vi "AutonomousChoose Postion.vi"() -> ()   [LabVIEW 2017]
doc: "This VI starts when autonomous period begins, and will automatically be terminated when it ends. You can carry out timed or sensor driven operations directly to I/O or to subsystems without needing to return to the caller."
uses:
  <vilib>/Rock Robotics/Network Tables/NT Read String.vi
panel:
  out "HandsMotorCmd":dbl(graph)
  out "Waveform Chart 4":u32(graph)
  out "millisecond timer value 2":u32
  out "SqueezeMotorCmd":dbl(graph)
  out "Lift Min Limit":bool
  out "Lift Max Limit":bool
  out "LiftMotorCmd":dbl(graph)
  out "Left Arm Max Limit":bool
  out "Right Arm Max Limit":bool
  out "Right Arm Min Limit":bool
  out "Left Arm Min Limit":bool
  out "LeftArmMotorCmd":dbl(graph)
  out "RightArmMotorCmd":dbl(graph)
  out "Arm Lift Min Limit":bool
  out "Arm Lift Max Limit":bool
  out "ArmLiftMotorCmd":dbl(graph)
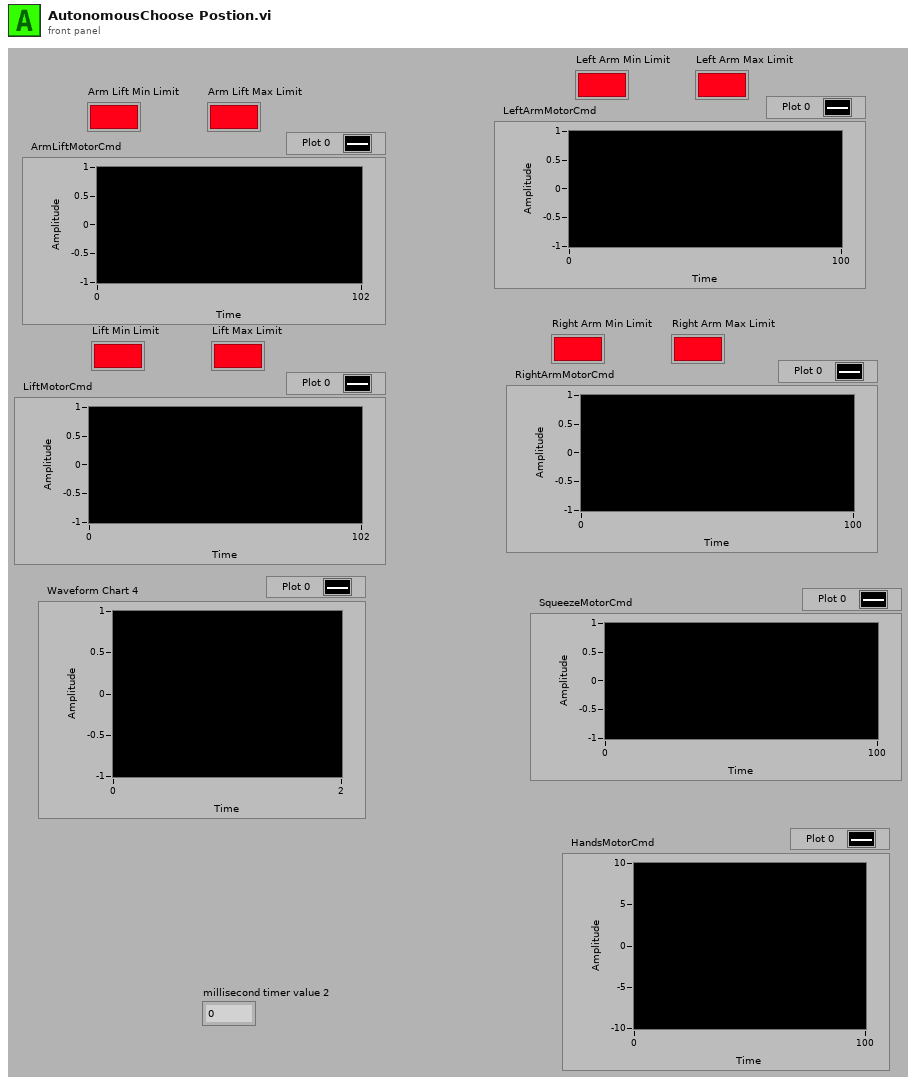
[diagram p1: front panel]
types:
  T1 = cluster{"X_axis":dbl, "Y_axis":dbl, "RotationTarget":dbl, "ArmLift":dbl, "Hands":dbl, "Lift":dbl, "Arms":dbl, "Squeeze":dbl}
  T2 = enum16{"initialize", "read", "write", "write all"}
  T3 = typedef "DioDisplayALB.ctl" = cluster{"DIO 0-LiftMinLimitSwitch":bool, "DIO 1-LiftMaxLimitSwitch":bool, "DIO 2-LiftArmMinLimitSwitch":bool, "DIO 3-LiftArmMaxLimitSwitch":bool, "DIO 4-RightArmMaxLimitSwitch":bool, "DIO 5-RightArmMinLimitSwitch":bool, "DIO 6-LeftArmMaxLimitSwitch":bool, "DIO 7-LeftArmMinLimitSwitch":bool, "DIO 8":bool, "DIO 9":bool}
  T4 = typedef "WPI_MotorControlDeviceRef.ctl" = cluster{"DeviceStatus":errorcluster, "Type":T5, "PWM":cluster{"PWM Channel":T6, "DeadBand":T7}, "CAN":cluster{"Device Number":u8, "SetOutput VI Ref":variant, "GetOutput VI Ref":variant, "Enable VI Ref":variant, "Disable VI Ref":variant, "Data":variant}, "Invert":bool, "DIO PWM":cluster{"PWM \"Enable\" Channel":T6, "DIOChannel":T8, "PWM Rate":dbl}}
  T5 = typedef "WPI_MotorControlType.ctl" = enum16{"PWM", "CAN", "DIO PWM"}
  T6 = typedef "FPGA_DIOPWMChannel.ctl" = enum8{"PWM 0", "PWM 1", "PWM 2", "PWM 3", "PWM 4", "PWM 5", "PWM 6", "PWM 7", "PWM 8", "PWM 9", "PWM MXP 0", "PWM MXP 1", "PWM MXP 2", "PWM MXP 3", "PWM MXP 4", "PWM MXP 5", "PWM MXP 6", "PWM MXP 7", "PWM MXP 8", "PWM MXP 9", "Invalid"}
  T7 = typedef "WPI_PWMDeadband.ctl" = cluster{"Name":string, "maxPositivePwm":i32, "minPositivePwm":i32, "centerPwm":i32, "maxNegativePwm":i32, "minNegativePwm":i32, "angularRange":u16}
  T8 = typedef "FPGA_DIOChannel.ctl" = enum8{"DIO 0", "DIO 1", "DIO 2", "DIO 3", "DIO 4", "DIO 5", "DIO 6", "DIO 7", "DIO 8", "DIO 9", "DIO MXP 0", "DIO MXP 1", "DIO MXP 2", "DIO MXP 3", "DIO MXP 4", "DIO MXP 5", "DIO MXP 6", "DIO MXP 7", "DIO MXP 8", "DIO MXP 9", "DIO MXP 10", "DIO MXP 11", "DIO MXP 12", "DIO MXP 13", "DIO MXP 14", "DIO MXP 15", "SPI Port CS1", "SPI Port CS2", "SPI Port CS3", "SPI Port MISO", "SPI Port MOSI", "Invalid"}
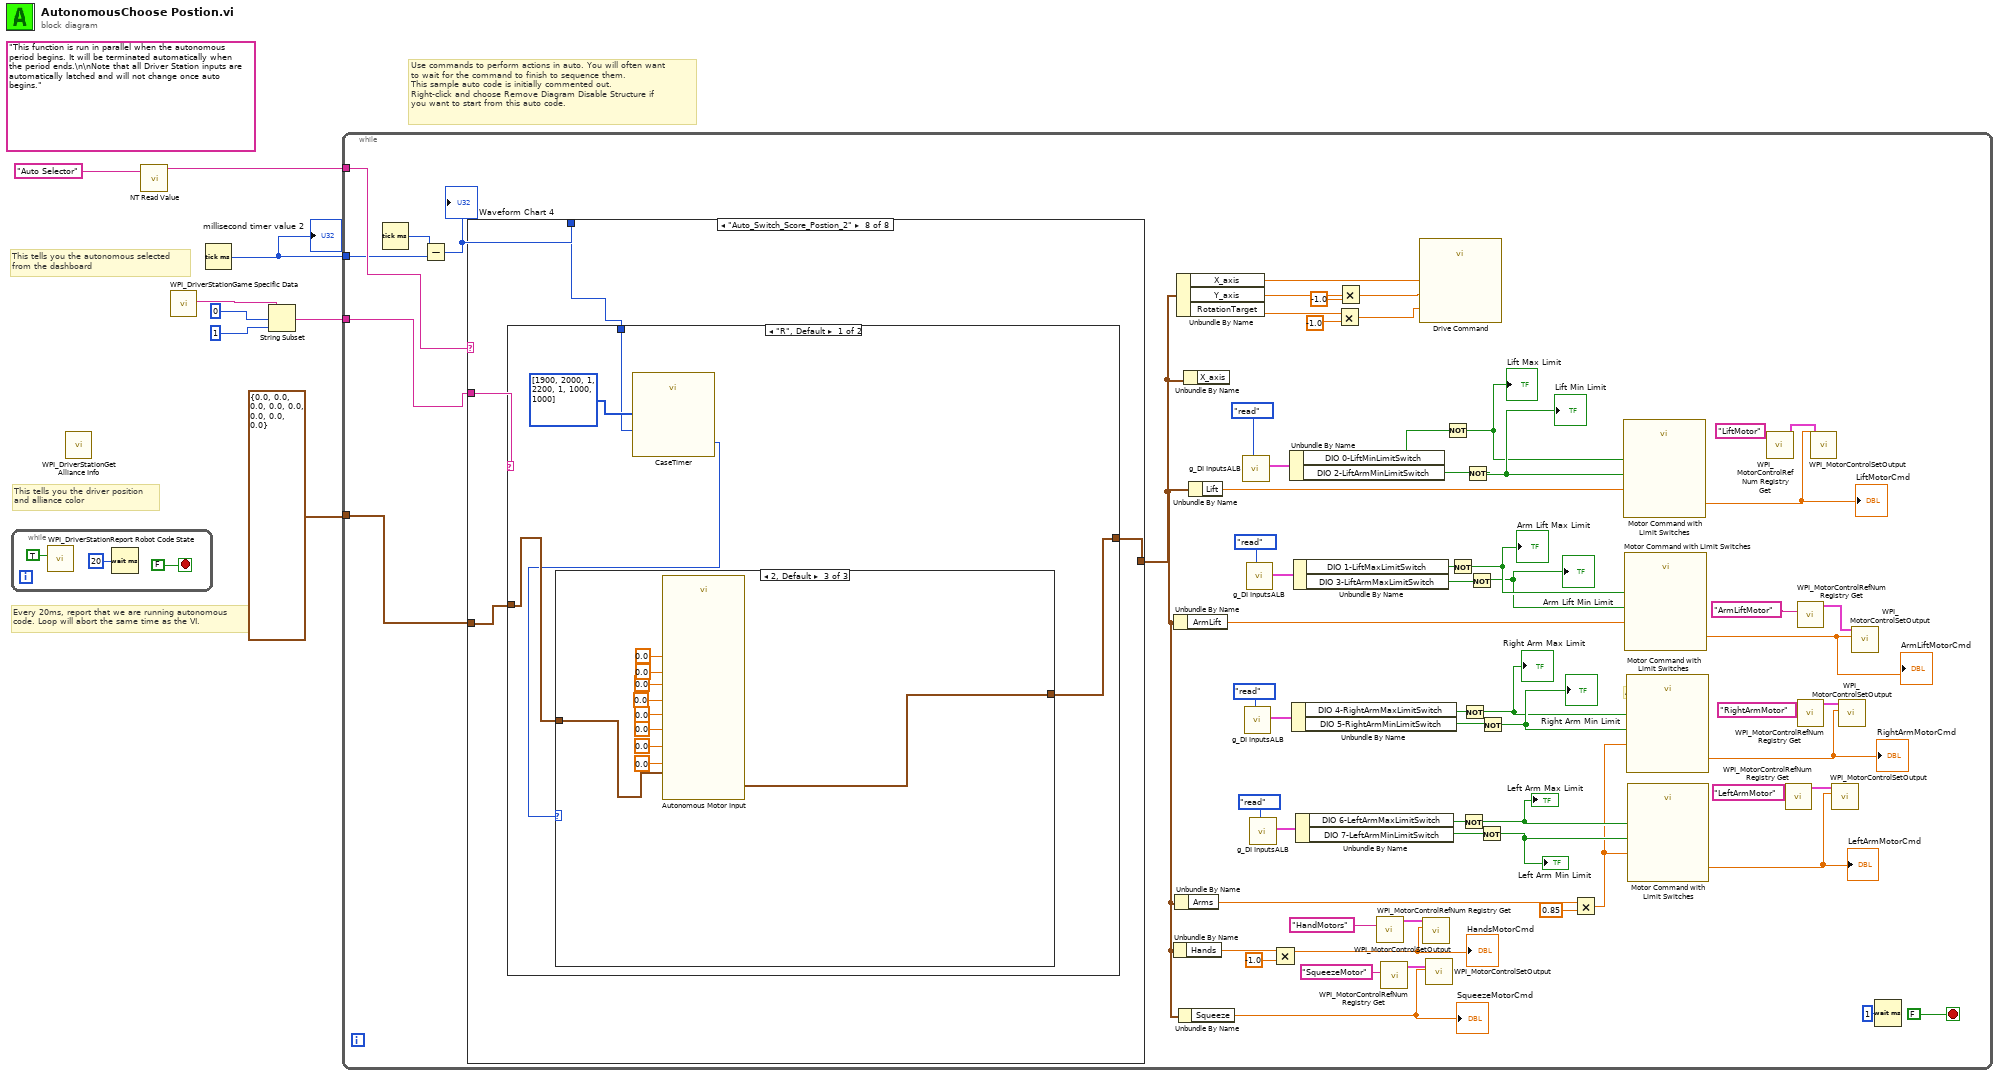
[diagram p0: block diagram]
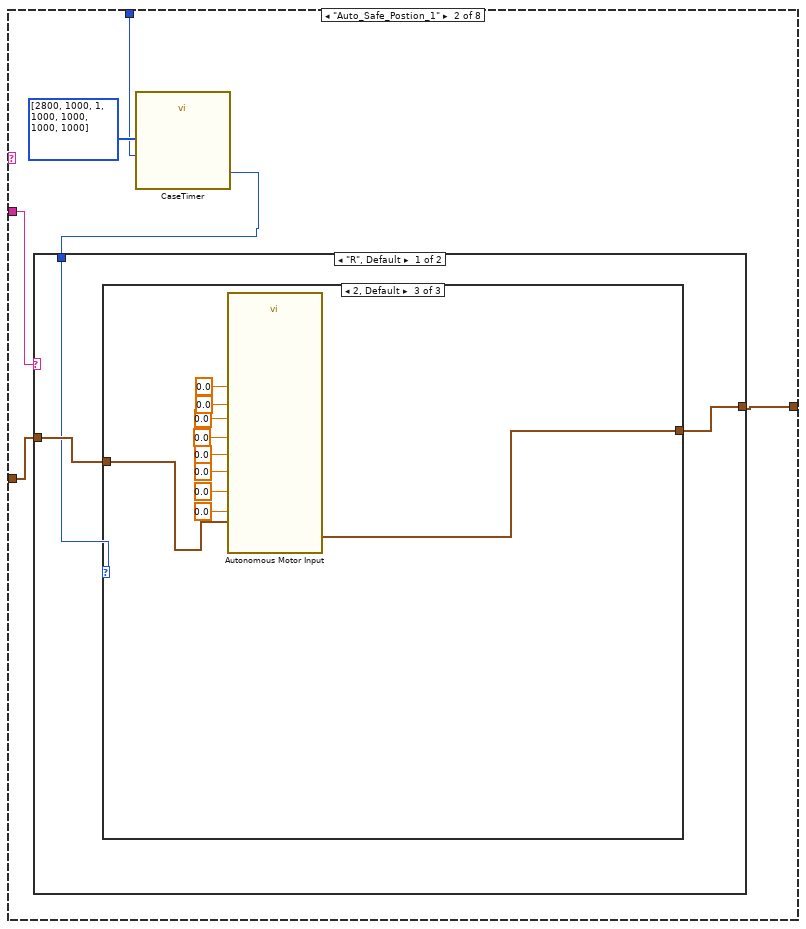
[diagram p3: hidden frame]
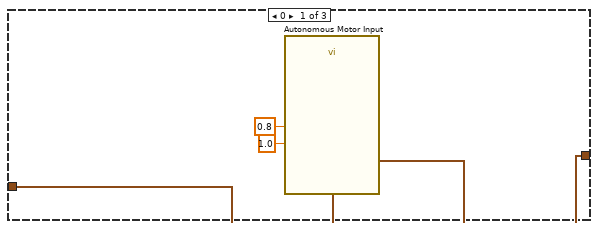
[diagram p4: hidden frame]
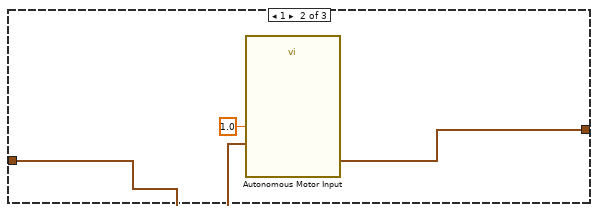
[diagram p5: hidden frame]
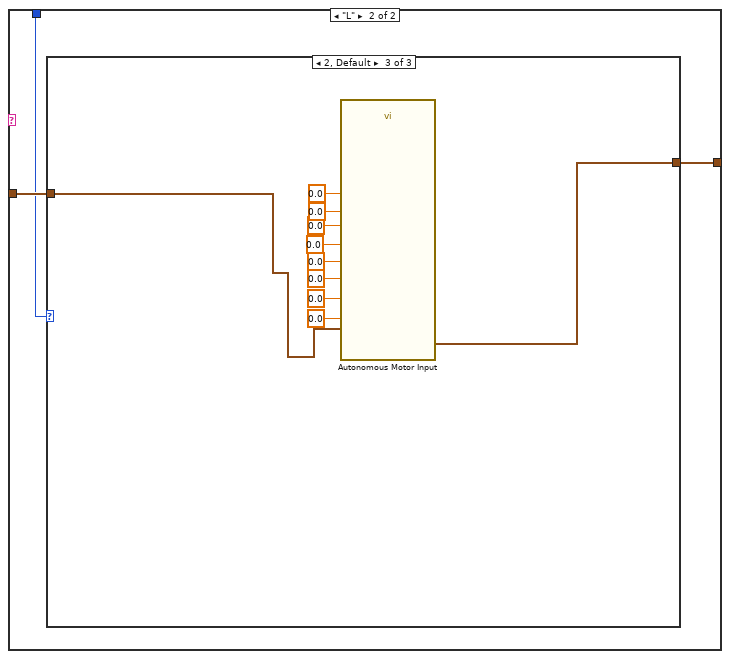
[diagram p6: hidden frame]
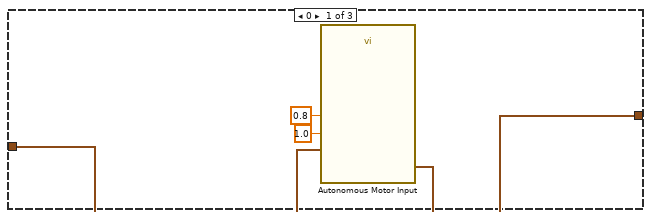
[diagram p7: hidden frame]
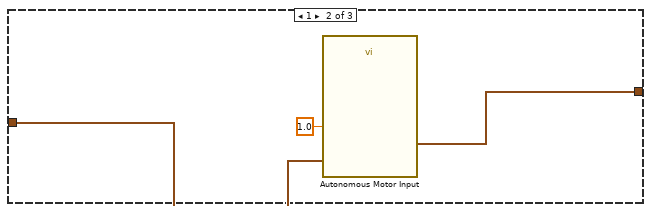
[diagram p8: hidden frame]
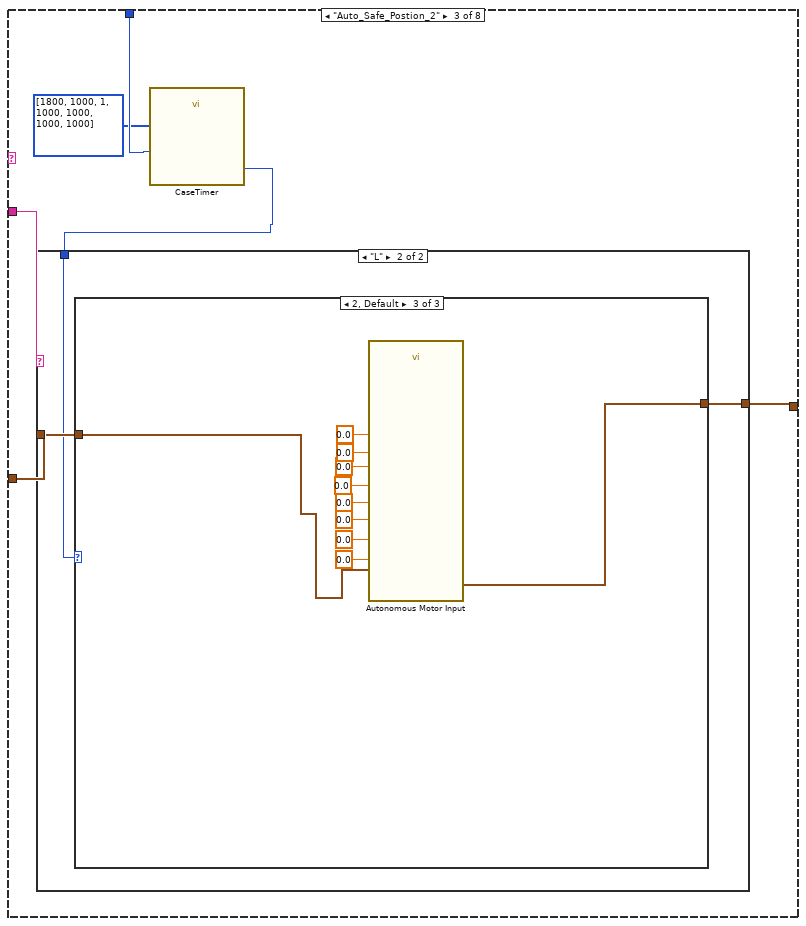
[diagram p9: hidden frame]
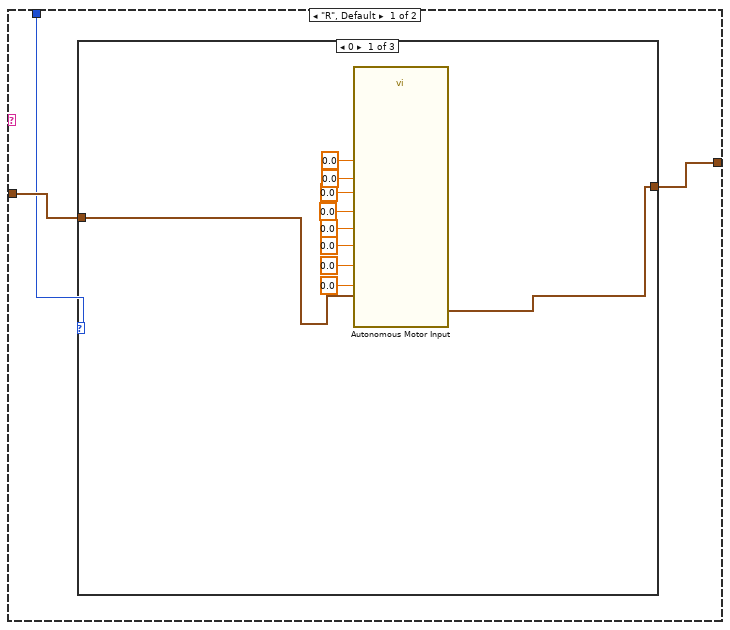
[diagram p10: hidden frame]
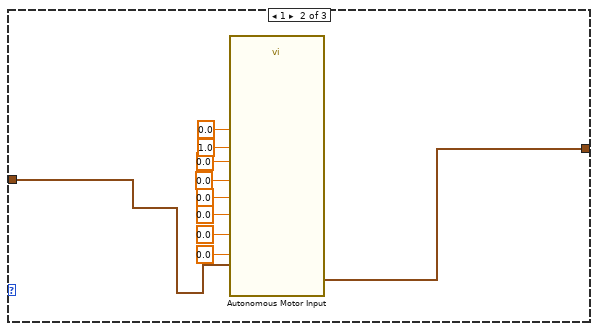
[diagram p11: hidden frame]
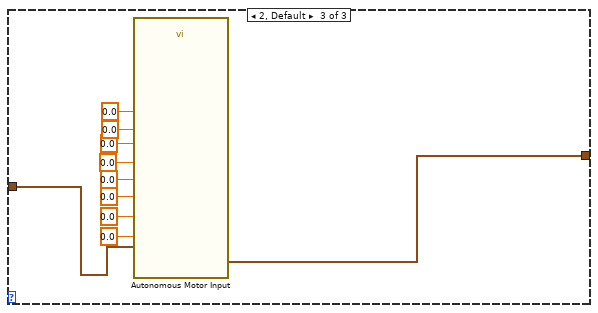
[diagram p12: hidden frame]
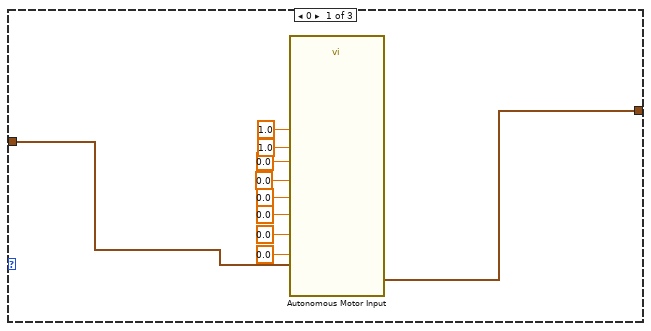
[diagram p13: hidden frame]
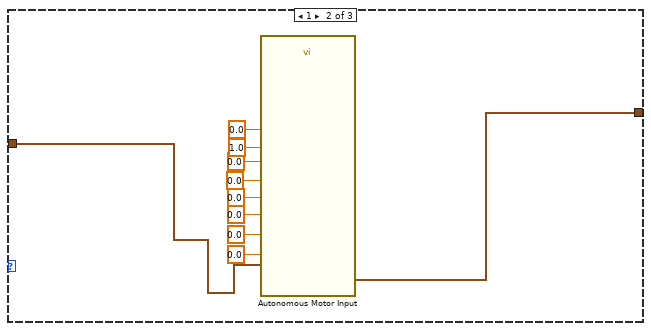
[diagram p14: hidden frame]
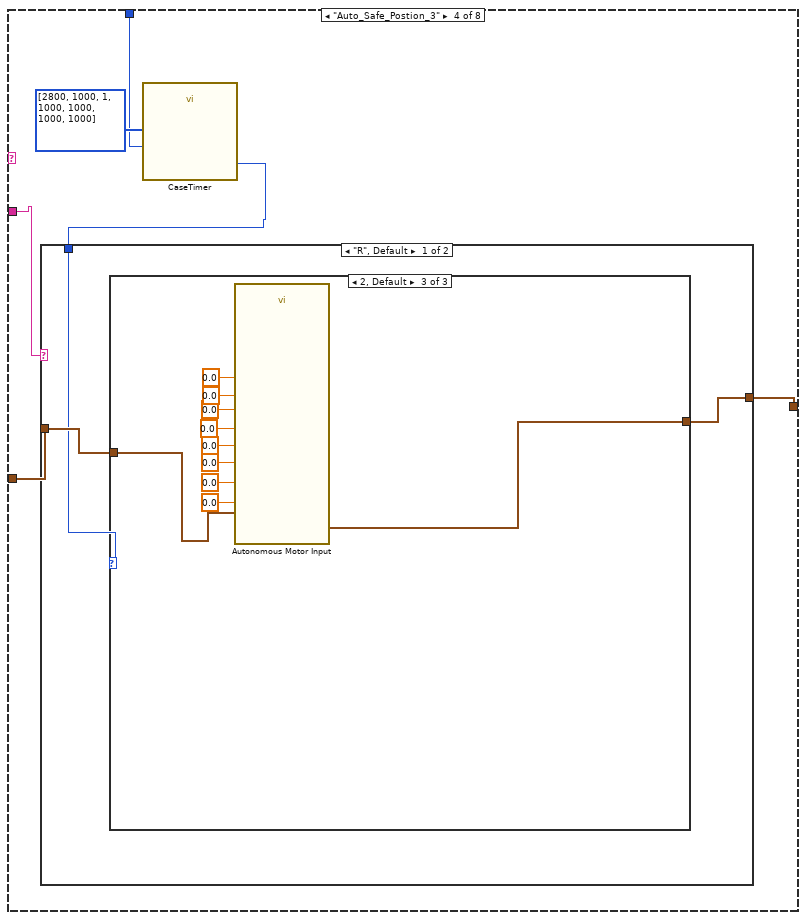
[diagram p15: hidden frame]
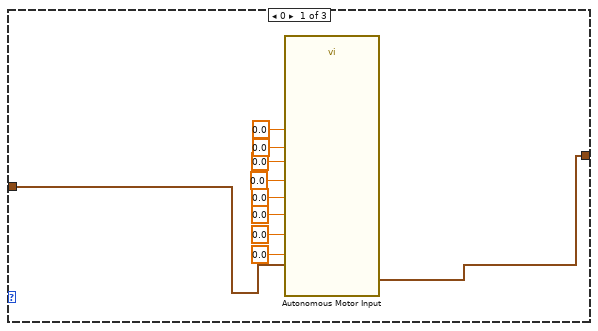
[diagram p16: hidden frame]
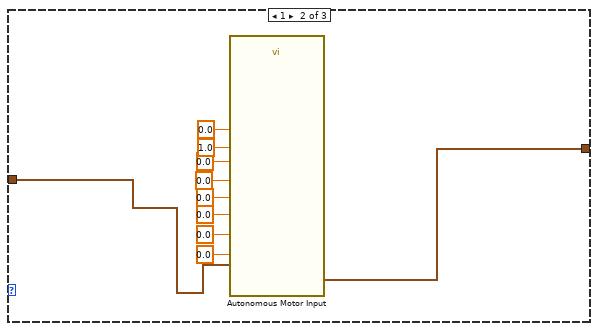
[diagram p17: hidden frame]
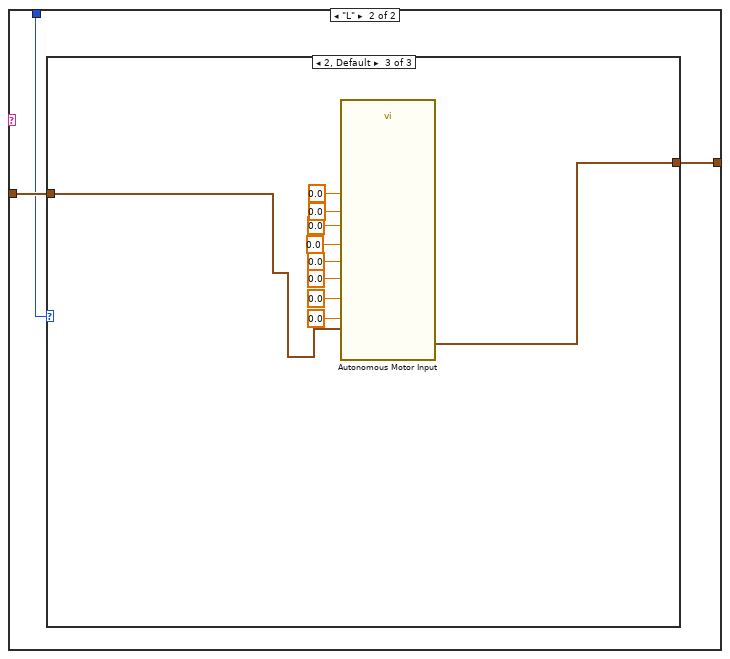
[diagram p18: hidden frame]
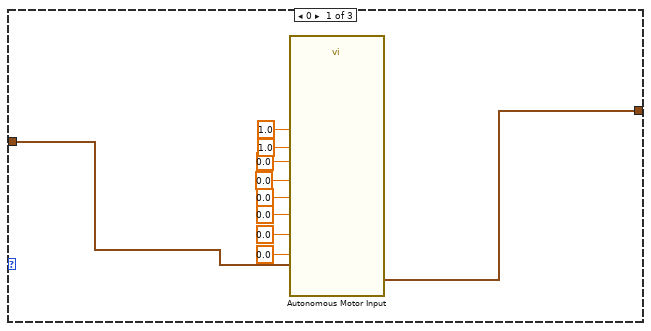
[diagram p19: hidden frame]
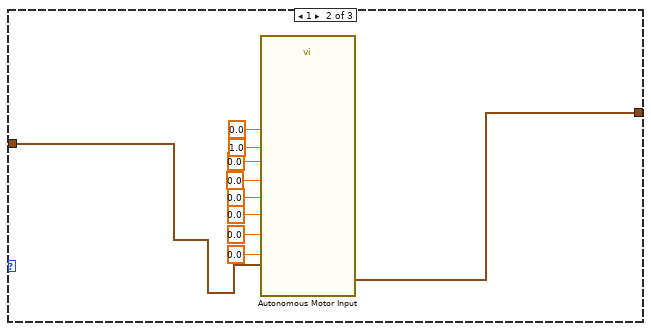
[diagram p20: hidden frame]
diagram:
  (unwired) "This function is run in parallel when the autonomous period begins. It will be terminated automatically when the period ends.\n\nNote that all Driver Station inputs are automatically latched and will not change once auto begins."
  # "This tells you the autonomous selected\nfrom the dashboard"
  # "Every 20ms, report that we are running autonomous\ncode. Loop will abort the same time as the VI."
  # "Use commands to perform actions in auto. You will often want\nto wait for the command to finish to sequence them.\nThis sample auto code is initially commented out. \nRight-click and choose Remove Diagram Disable Structure if\nyou want to start from this auto code."
  # "This tells you the driver position\nand alliance color"
  n1 = while {
    stop <- FALSE stop-if-true
    n2 = call <vilib>:"WPI_DriverStationReport Robot Code State.vi"("Autonomous"=TRUE) -> ()  [unwired: 10 in, 1 out]
    n3 = Wait (ms)(milliseconds to wait=u32 20) -> ()  [unwired: 1 out]
  }
  n4 = call <vilib>:"WPI_DriverStationGet Alliance Info.vi"() -> ()  [unwired: 12 out]
  n5 = call-poly <vilib>:"NT Read Value.vi"("Name"="Auto Selector") -> ("String"=w7:string)  [unwired: 9 in, 1 out]
  n6 = call <vilib>:"WPI_DriverStationGame Specific Data.vi"() -> ("Game Specific Data"=w4:string)  [unwired: 11 in]
  n7 = Tick Count (ms)() -> (millisecond timer value=w5:u32)
  "millisecond timer value 2" <- w5
  n8 = String Subset(string=w4, offset (0)=0, length (rest)=1 ("length (rest)")) -> (substring=w1:string)
  n9 = while {
    tunnel: w7 -> [w75]
    tunnel: T1 {"X_axis"=0.0, "Y_axis"=0.0, "RotationTarget"=0.0, "ArmLift"=0.0, "Hands"=0.0, "Lift"=0.0, "Arms"=0.0, "Squeeze"=0.0} ("Cluster") -> [w74]
    tunnel: w5 -> [w24]
    tunnel: w1 -> [w13]
    stop <- FALSE stop-if-true
    # "Arms"
    n10 = Tick Count (ms)() -> (millisecond timer value=w25:u32)
    n11 = Subtract(x=w25, y=w24) -> (x-y=w12:u32)
    "Waveform Chart 4" <- w12
    n12 = case shown="\"Auto_Switch_Score_Postion_2\"" w75 {
      tunnel: w74 -> [w77 w82 w128 w198 w269 w364 w413 w469]
      tunnel: [w77 w81 w126 w197 w271 w365 w412 w468] -> w26
      tunnel: w13 -> [_ w83 w127 w199 w270 w362 w414 w470]
      tunnel: w12 -> [_ w79 w125 w196 w268 w363 w411 w471]
      frame Default {
        # "You can put your main auto here, or you can right-click on the case and make any\nother frame be the default case."
        # "This is the frame that will execute if no selection is made, or if it is not recognized"
      }
      frame "Auto_Safe_Postion_1" {
        n13 = call "CaseTimer.vi"("CaseTime"=u32[] [2800, 1000, 1, 1000, 1000, 1000, 1000], "ElapsedTime"=w79) -> ("CaseNumber"=w78:i32)  [unwired: 9 in]
        n14 = case shown="\"R\", Default" w83 {
          tunnel: w82 -> [w86 w106]
          tunnel: [w85 w105] -> w81
          tunnel: w78 -> [w84 w104]
          frame "R", Default {
            n15 = case shown="2, Default" w84 {
              tunnel: w86 -> [w90 w93 w96]
              tunnel: [w89 w92 w94] -> w85
              frame 0 {
                n16 = call "Autonomous Motor Input.vi"("Y_axis"=0.8, "Cluster in"=w90, "Arms"=1.0) -> ("Cluster out"=w89:T1)  [unwired: 12 in]
              }
              frame 1 {
                n17 = call "Autonomous Motor Input.vi"("Cluster in"=w93, "Arms"=1.0) -> ("Cluster out"=w92:T1)  [unwired: 13 in]
              }
              frame 2, Default {
                n18 = call "Autonomous Motor Input.vi"("RotationTarget"=0.0, "Y_axis"=0.0, "X_axis"=0.0, "Squeeze"=0.0, "Cluster in"=w96, "Arms"=0.0, "ArmLift"=0.0, "Hands"=0.0, "Lift"=0.0) -> ("Cluster out"=w94:T1)  [unwired: 6 in]
              }
            }
          }
          frame "L" {
            n19 = case shown="2, Default" w104 {
              tunnel: w106 -> [w110 w113 w115]
              tunnel: [w109 w112 w114] -> w105
              frame 0 {
                n20 = call "Autonomous Motor Input.vi"("Y_axis"=0.8, "Cluster in"=w110, "Arms"=1.0) -> ("Cluster out"=w109:T1)  [unwired: 12 in]
              }
              frame 1 {
                n21 = call "Autonomous Motor Input.vi"("Cluster in"=w113, "Arms"=1.0) -> ("Cluster out"=w112:T1)  [unwired: 13 in]
              }
              frame 2, Default {
                n22 = call "Autonomous Motor Input.vi"("RotationTarget"=0.0, "Y_axis"=0.0, "X_axis"=0.0, "Squeeze"=0.0, "Cluster in"=w115, "Arms"=0.0, "ArmLift"=0.0, "Hands"=0.0, "Lift"=0.0) -> ("Cluster out"=w114:T1)  [unwired: 6 in]
              }
            }
          }
        }
      }
      frame "Auto_Safe_Postion_2" {
        n23 = call "CaseTimer.vi"("CaseTime"=u32[] [1800, 1000, 1, 1000, 1000, 1000, 1000], "ElapsedTime"=w125) -> ("CaseNumber"=w129:i32)  [unwired: 9 in]
        n24 = case shown="\"L\"" w127 {
          tunnel: w128 -> [w132 w165]
          tunnel: [w131 w164] -> w126
          tunnel: w129 -> [w130 w163]
          frame "R", Default {
            n25 = case shown="0" w130 {
              tunnel: w132 -> [w134 w144 w155]
              tunnel: [w133 w143 w153] -> w131
              frame 0 {
                n26 = call "Autonomous Motor Input.vi"("RotationTarget"=0.0, "Y_axis"=0.0, "X_axis"=0.0, "Squeeze"=0.0, "Cluster in"=w134, "Arms"=0.0, "ArmLift"=0.0, "Hands"=0.0, "Lift"=0.0) -> ("Cluster out"=w133:T1)  [unwired: 6 in]
              }
              frame 1 {
                n27 = call "Autonomous Motor Input.vi"("RotationTarget"=0.0, "Y_axis"=0.0, "X_axis"=0.0, "Squeeze"=0.0, "Cluster in"=w144, "Arms"=1.0, "ArmLift"=0.0, "Hands"=0.0, "Lift"=0.0) -> ("Cluster out"=w143:T1)  [unwired: 6 in]
              }
              frame 2, Default {
                n28 = call "Autonomous Motor Input.vi"("RotationTarget"=0.0, "Y_axis"=0.0, "X_axis"=0.0, "Squeeze"=0.0, "Cluster in"=w155, "Arms"=0.0, "ArmLift"=0.0, "Hands"=0.0, "Lift"=0.0) -> ("Cluster out"=w153:T1)  [unwired: 6 in]
              }
            }
          }
          frame "L" {
            n29 = case shown="2, Default" w163 {
              tunnel: w165 -> [w167 w177 w187]
              tunnel: [w166 w176 w186] -> w164
              frame 0 {
                n30 = call "Autonomous Motor Input.vi"("RotationTarget"=0.0, "Y_axis"=1.0, "X_axis"=0.0, "Squeeze"=0.0, "Cluster in"=w167, "Arms"=1.0, "ArmLift"=0.0, "Hands"=0.0, "Lift"=0.0) -> ("Cluster out"=w166:T1)  [unwired: 6 in]
              }
              frame 1 {
                n31 = call "Autonomous Motor Input.vi"("RotationTarget"=0.0, "Y_axis"=0.0, "X_axis"=0.0, "Squeeze"=0.0, "Cluster in"=w177, "Arms"=1.0, "ArmLift"=0.0, "Hands"=0.0, "Lift"=0.0) -> ("Cluster out"=w176:T1)  [unwired: 6 in]
              }
              frame 2, Default {
                n32 = call "Autonomous Motor Input.vi"("RotationTarget"=0.0, "Y_axis"=0.0, "X_axis"=0.0, "Squeeze"=0.0, "Cluster in"=w187, "Arms"=0.0, "ArmLift"=0.0, "Hands"=0.0, "Lift"=0.0) -> ("Cluster out"=w186:T1)  [unwired: 6 in]
              }
            }
          }
        }
      }
      frame "Auto_Safe_Postion_3" {
        n33 = call "CaseTimer.vi"("CaseTime"=u32[] [2800, 1000, 1, 1000, 1000, 1000, 1000], "ElapsedTime"=w196) -> ("CaseNumber"=w200:i32)  [unwired: 9 in]
        n34 = case shown="\"R\", Default" w199 {
          tunnel: w198 -> [w204 w237]
          tunnel: [w203 w236] -> w197
          tunnel: w200 -> [w202 w235]
          frame "R", Default {
            n35 = case shown="2, Default" w202 {
              tunnel: w204 -> [w206 w216 w227]
              tunnel: [w205 w215 w225] -> w203
              frame 0 {
                n36 = call "Autonomous Motor Input.vi"("RotationTarget"=0.0, "Y_axis"=0.0, "X_axis"=0.0, "Squeeze"=0.0, "Cluster in"=w206, "Arms"=0.0, "ArmLift"=0.0, "Hands"=0.0, "Lift"=0.0) -> ("Cluster out"=w205:T1)  [unwired: 6 in]
              }
              frame 1 {
                n37 = call "Autonomous Motor Input.vi"("RotationTarget"=0.0, "Y_axis"=0.0, "X_axis"=0.0, "Squeeze"=0.0, "Cluster in"=w216, "Arms"=1.0, "ArmLift"=0.0, "Hands"=0.0, "Lift"=0.0) -> ("Cluster out"=w215:T1)  [unwired: 6 in]
              }
              frame 2, Default {
                n38 = call "Autonomous Motor Input.vi"("RotationTarget"=0.0, "Y_axis"=0.0, "X_axis"=0.0, "Squeeze"=0.0, "Cluster in"=w227, "Arms"=0.0, "ArmLift"=0.0, "Hands"=0.0, "Lift"=0.0) -> ("Cluster out"=w225:T1)  [unwired: 6 in]
              }
            }
          }
          frame "L" {
            n39 = case shown="2, Default" w235 {
              tunnel: w237 -> [w239 w249 w259]
              tunnel: [w238 w248 w258] -> w236
              frame 0 {
                n40 = call "Autonomous Motor Input.vi"("RotationTarget"=0.0, "Y_axis"=1.0, "X_axis"=0.0, "Squeeze"=0.0, "Cluster in"=w239, "Arms"=1.0, "ArmLift"=0.0, "Hands"=0.0, "Lift"=0.0) -> ("Cluster out"=w238:T1)  [unwired: 6 in]
              }
              frame 1 {
                n41 = call "Autonomous Motor Input.vi"("RotationTarget"=0.0, "Y_axis"=0.0, "X_axis"=0.0, "Squeeze"=0.0, "Cluster in"=w249, "Arms"=1.0, "ArmLift"=0.0, "Hands"=0.0, "Lift"=0.0) -> ("Cluster out"=w248:T1)  [unwired: 6 in]
              }
              frame 2, Default {
                n42 = call "Autonomous Motor Input.vi"("RotationTarget"=0.0, "Y_axis"=0.0, "X_axis"=0.0, "Squeeze"=0.0, "Cluster in"=w259, "Arms"=0.0, "ArmLift"=0.0, "Hands"=0.0, "Lift"=0.0) -> ("Cluster out"=w258:T1)  [unwired: 6 in]
              }
            }
          }
        }
      }
      frame "Auto_Switch_Postion_1" {
        n43 = case shown="\"R\", Default" w270 {
          tunnel: [w276 w311] -> w271
          tunnel: w269 -> [w275 w310]
          tunnel: w268 -> [w273 w308]
          frame "R", Default {
            n44 = call "CaseTimer.vi"("CaseTime"=u32[] [2800, 2000, 1, 2200, 1, 1000, 1000], "ElapsedTime"=w273) -> ("CaseNumber"=w272:i32)  [unwired: 9 in]
            n45 = case shown="2, Default" w272 {
              tunnel: w275 -> [w278 w288 w299]
              tunnel: [w277 w287 w297] -> w276
              frame 0 {
                n46 = call "Autonomous Motor Input.vi"("RotationTarget"=0.0, "Y_axis"=1.0, "X_axis"=0.0, "Squeeze"=0.0, "Cluster in"=w278, "Arms"=1.0, "ArmLift"=0.0, "Hands"=0.0, "Lift"=0.0) -> ("Cluster out"=w277:T1)  [unwired: 6 in]
              }
              frame 1 {
                n47 = call "Autonomous Motor Input.vi"("RotationTarget"=0.0, "Y_axis"=0.0, "X_axis"=0.0, "Squeeze"=0.0, "Cluster in"=w288, "Arms"=1.0, "ArmLift"=0.0, "Hands"=0.0, "Lift"=0.0) -> ("Cluster out"=w287:T1)  [unwired: 6 in]
              }
              frame 2, Default {
                n48 = call "Autonomous Motor Input.vi"("RotationTarget"=0.0, "Y_axis"=0.0, "X_axis"=0.0, "Squeeze"=0.0, "Cluster in"=w299, "Arms"=0.0, "ArmLift"=0.0, "Hands"=0.0, "Lift"=0.0) -> ("Cluster out"=w297:T1)  [unwired: 6 in]
              }
            }
          }
          frame "L" {
            n49 = call "CaseTimer.vi"("CaseTime"=u32[] [2800, 660, 400, 2200, 1, 1000, 1000], "ElapsedTime"=w308) -> ("CaseNumber"=w307:i32)  [unwired: 9 in]
            n50 = case shown="0" w307 {
              tunnel: w310 -> [w313 w323 w333 w343 w353]
              tunnel: [w312 w322 w332 w342 w352] -> w311
              frame 0 {
                n51 = call "Autonomous Motor Input.vi"("RotationTarget"=0.0, "Y_axis"=0.8, "X_axis"=0.0, "Squeeze"=0.0, "Cluster in"=w313, "Arms"=1.0, "ArmLift"=0.0, "Hands"=0.0, "Lift"=0.0) -> ("Cluster out"=w312:T1)  [unwired: 6 in]
              }
              frame 1 {
                n52 = call "Autonomous Motor Input.vi"("RotationTarget"=0.0, "Y_axis"=0.0, "X_axis"=1.0, "Squeeze"=0.0, "Cluster in"=w323, "Arms"=1.0, "ArmLift"=0.0, "Hands"=0.0, "Lift"=0.0) -> ("Cluster out"=w322:T1)  [unwired: 6 in]
              }
              frame 2 {
                n53 = call "Autonomous Motor Input.vi"("RotationTarget"=0.0, "Y_axis"=1.0, "X_axis"=0.0, "Squeeze"=0.0, "Cluster in"=w333, "Arms"=1.0, "ArmLift"=0.0, "Hands"=0.0, "Lift"=0.0) -> ("Cluster out"=w332:T1)  [unwired: 6 in]
              }
              frame 3 {
                n54 = call "Autonomous Motor Input.vi"("RotationTarget"=0.0, "Y_axis"=0.0, "X_axis"=0.0, "Squeeze"=0.0, "Cluster in"=w343, "Arms"=1.0, "ArmLift"=0.0, "Hands"=1.0, "Lift"=0.0) -> ("Cluster out"=w342:T1)  [unwired: 6 in]
              }
              frame 4, Default {
                n55 = call "Autonomous Motor Input.vi"("RotationTarget"=0.0, "Y_axis"=0.0, "X_axis"=0.0, "Squeeze"=0.0, "Cluster in"=w353, "Arms"=0.0, "ArmLift"=0.0, "Hands"=0.0, "Lift"=0.0) -> ("Cluster out"=w352:T1)  [unwired: 6 in]
              }
            }
          }
        }
      }
      frame "Auto_Switch_Postion_2" {
        n56 = case shown="\"R\", Default" w362 {
          tunnel: [w370 w393] -> w365
          tunnel: w364 -> [w369 w392]
          tunnel: w363 -> [w367 w390]
          frame "R", Default {
            n57 = call "CaseTimer.vi"("CaseTime"=u32[] [1900, 2000, 1, 2200, 1, 1000, 1000], "ElapsedTime"=w367) -> ("CaseNumber"=w366:i32)  [unwired: 9 in]
            n58 = case shown="1" w366 {
              tunnel: w369 -> [w374 w378 w381]
              tunnel: [w373 w377 w379] -> w370
              frame 0 {
                n59 = call "Autonomous Motor Input.vi"("Y_axis"=0.9, "Cluster in"=w374, "Arms"=1.0) -> ("Cluster out"=w373:T1)  [unwired: 12 in]
              }
              frame 1 {
                n60 = call "Autonomous Motor Input.vi"("Cluster in"=w378, "Arms"=1.0, "Hands"=1.0) -> ("Cluster out"=w377:T1)  [unwired: 12 in]
              }
              frame 2, Default {
                n61 = call "Autonomous Motor Input.vi"("RotationTarget"=0.0, "Y_axis"=0.0, "X_axis"=0.0, "Squeeze"=0.0, "Cluster in"=w381, "Arms"=0.0, "ArmLift"=0.0, "Hands"=0.0, "Lift"=0.0) -> ("Cluster out"=w379:T1)  [unwired: 6 in]
              }
            }
          }
          frame "L" {
            n62 = call "CaseTimer.vi"("CaseTime"=u32[] [1800, 2500, 1, 2200, 1, 1000, 1000], "ElapsedTime"=w390) -> ("CaseNumber"=w389:i32)  [unwired: 9 in]
            n63 = case shown="2, Default" w389 {
              tunnel: w392 -> [w397 w400 w402]
              tunnel: [w396 w399 w401] -> w393
              frame 0 {
                n64 = call "Autonomous Motor Input.vi"("Y_axis"=0.9, "Cluster in"=w397, "Arms"=1.0) -> ("Cluster out"=w396:T1)  [unwired: 12 in]
              }
              frame 1 {
                n65 = call "Autonomous Motor Input.vi"("Cluster in"=w400, "Arms"=1.0) -> ("Cluster out"=w399:T1)  [unwired: 13 in]
              }
              frame 2, Default {
                n66 = call "Autonomous Motor Input.vi"("RotationTarget"=0.0, "Y_axis"=0.0, "X_axis"=0.0, "Squeeze"=0.0, "Cluster in"=w402, "Arms"=0.0, "ArmLift"=0.0, "Hands"=0.0, "Lift"=0.0) -> ("Cluster out"=w401:T1)  [unwired: 6 in]
              }
            }
          }
        }
      }
      frame "Auto_Switch_Postion_3" {
        n67 = case shown="\"R\", Default" w414 {
          tunnel: [w419 w450] -> w412
          tunnel: w413 -> [w418 w449]
          tunnel: w411 -> [w416 w447]
          frame "R", Default {
            n68 = call "CaseTimer.vi"("CaseTime"=u32[] [2800, 660, 400, 2200, 1, 1000, 1000], "ElapsedTime"=w416) -> ("CaseNumber"=w415:i32)  [unwired: 9 in]
            n69 = case shown="3" w415 {
              tunnel: w418 -> [w423 w427 w430 w435 w438]
              tunnel: [w422 w426 w429 w434 w436] -> w419
              frame 0 {
                n70 = call "Autonomous Motor Input.vi"("Y_axis"=1.0, "Cluster in"=w423, "Arms"=1.0) -> ("Cluster out"=w422:T1)  [unwired: 12 in]
              }
              frame 1 {
                n71 = call "Autonomous Motor Input.vi"("X_axis"=-1.0 ("Hands"), "Cluster in"=w427, "Arms"=1.0) -> ("Cluster out"=w426:T1)  [unwired: 12 in]
              }
              frame 2 {
                n72 = call "Autonomous Motor Input.vi"("Y_axis"=1.0 ("Hands"), "Cluster in"=w430, "Arms"=1.0) -> ("Cluster out"=w429:T1)  [unwired: 12 in]
              }
              frame 3 {
                n73 = call "Autonomous Motor Input.vi"("Cluster in"=w435, "Arms"=1.0, "Hands"=1.0) -> ("Cluster out"=w434:T1)  [unwired: 12 in]
              }
              frame 4, Default {
                n74 = call "Autonomous Motor Input.vi"("RotationTarget"=0.0, "Y_axis"=0.0, "X_axis"=0.0, "Squeeze"=0.0, "Cluster in"=w438, "Arms"=0.0, "ArmLift"=0.0, "Hands"=0.0, "Lift"=0.0) -> ("Cluster out"=w436:T1)  [unwired: 6 in]
              }
            }
          }
          frame "L" {
            n75 = call "CaseTimer.vi"("CaseTime"=u32[] [2800, 2500, 1, 2200, 1, 1000, 1000], "ElapsedTime"=w447) -> ("CaseNumber"=w446:i32)  [unwired: 9 in]
            n76 = case shown="1" w446 {
              tunnel: w449 -> [w454 w457 w459]
              tunnel: [w453 w456 w458] -> w450
              frame 0 {
                n77 = call "Autonomous Motor Input.vi"("Y_axis"=1.0, "Cluster in"=w454, "Arms"=1.0) -> ("Cluster out"=w453:T1)  [unwired: 12 in]
              }
              frame 1 {
                n78 = call "Autonomous Motor Input.vi"("Cluster in"=w457, "Arms"=1.0) -> ("Cluster out"=w456:T1)  [unwired: 13 in]
              }
              frame 2, Default {
                n79 = call "Autonomous Motor Input.vi"("RotationTarget"=0.0, "Y_axis"=0.0, "X_axis"=0.0, "Squeeze"=0.0, "Cluster in"=w459, "Arms"=0.0, "ArmLift"=0.0, "Hands"=0.0, "Lift"=0.0) -> ("Cluster out"=w458:T1)  [unwired: 6 in]
              }
            }
          }
        }
      }
      frame "Auto_Switch_Score_Postion_2" {
        n80 = case shown="\"R\", Default" w470 {
          tunnel: [w476 w499] -> w468
          tunnel: w469 -> [w475 w498]
          tunnel: w471 -> [w473 w496]
          frame "R", Default {
            n81 = call "CaseTimer.vi"("CaseTime"=u32[] [1900, 2000, 1, 2200, 1, 1000, 1000], "ElapsedTime"=w473) -> ("CaseNumber"=w472:i32)  [unwired: 9 in]
            n82 = case shown="2, Default" w472 {
              tunnel: w475 -> [w480 w484 w487]
              tunnel: [w479 w483 w485] -> w476
              frame 0 {
                n83 = call "Autonomous Motor Input.vi"("Y_axis"=0.9, "Cluster in"=w480, "Arms"=1.0) -> ("Cluster out"=w479:T1)  [unwired: 12 in]
              }
              frame 1 {
                n84 = call "Autonomous Motor Input.vi"("Cluster in"=w484, "Arms"=1.0, "Hands"=1.0) -> ("Cluster out"=w483:T1)  [unwired: 12 in]
              }
              frame 2, Default {
                n85 = call "Autonomous Motor Input.vi"("RotationTarget"=0.0, "Y_axis"=0.0, "X_axis"=0.0, "Squeeze"=0.0, "Cluster in"=w487, "Arms"=0.0, "ArmLift"=0.0, "Hands"=0.0, "Lift"=0.0) -> ("Cluster out"=w485:T1)  [unwired: 6 in]
              }
            }
          }
          frame "L" {
            n86 = call "CaseTimer.vi"("CaseTime"=u32[] [800, 660, 1000, 660, 900, 1000, 1], "ElapsedTime"=w496) -> ("CaseNumber"=w495:i32)  [unwired: 9 in]
            n87 = case shown="6, Default" w495 {
              tunnel: w498 -> [w503 w507 w510 w514 w518 w522 w524]
              tunnel: [w502 w506 w509 w513 w517 w521 w523] -> w499
              frame 0 {
                n88 = call "Autonomous Motor Input.vi"("Y_axis"=0.9, "Cluster in"=w503, "Arms"=1.0) -> ("Cluster out"=w502:T1)  [unwired: 12 in]
              }
              frame 1 {
                n89 = call "Autonomous Motor Input.vi"("X_axis"=-1.0, "Cluster in"=w507, "Arms"=1.0) -> ("Cluster out"=w506:T1)  [unwired: 12 in]
              }
              frame 2 {
                n90 = call "Autonomous Motor Input.vi"("Y_axis"=0.5, "Cluster in"=w510) -> ("Cluster out"=w509:T1)  [unwired: 13 in]
              }
              frame 3 {
                n91 = call "Autonomous Motor Input.vi"("X_axis"=1.0, "Cluster in"=w514, "Arms"=1.0) -> ("Cluster out"=w513:T1)  [unwired: 12 in]
              }
              frame 4 {
                n92 = call "Autonomous Motor Input.vi"("Y_axis"=1.0, "Cluster in"=w518, "Arms"=1.0) -> ("Cluster out"=w517:T1)  [unwired: 12 in]
              }
              frame 5 {
                n93 = call "Autonomous Motor Input.vi"("Cluster in"=w522, "Arms"=1.0, "Hands"=1.0) -> ("Cluster out"=w521:T1)  [unwired: 12 in]
              }
              frame 6, Default {
                n94 = call "Autonomous Motor Input.vi"("RotationTarget"=0.0, "Y_axis"=0.0, "X_axis"=0.0, "Squeeze"=0.0, "Cluster in"=w524, "Arms"=0.0, "ArmLift"=0.0, "Hands"=0.0, "Lift"=0.0) -> ("Cluster out"=w523:T1)  [unwired: 6 in]
              }
            }
          }
        }
      }
    }
    n95 = Unbundle By Name(w26) -> ("Hands"=w20:dbl)
    n96 = Unbundle By Name(w26) -> ("ArmLift"=w60:dbl)
    n97 = Unbundle By Name(w26) -> ("Arms"=w39:dbl)
    n98 = Unbundle By Name(w26) -> ("X_axis"=w72:dbl, "Y_axis"=w23:dbl, "RotationTarget"=w18:dbl)
    n99 = Unbundle By Name(w26) -> ("Squeeze"=w27:dbl)
    "SqueezeMotorCmd" <- w27
    n100 = Unbundle By Name(w26) -> ()  [unwired: 1 out]
    n101 = Unbundle By Name(w26) -> ("Lift"=w29:dbl)
    n102 = call "g_DI InputsALB.vi"("Action"=T2."read") -> ("DI out"=w33:T3)  [unwired: 10 in]
    n103 = call "g_DI InputsALB.vi"("Action"=T2."read") -> ("DI out"=w42:T3)  [unwired: 10 in]
    n104 = call "g_DI InputsALB.vi"("Action"=T2."read") -> ("DI out"=w64:T3)  [unwired: 10 in]
    n105 = call "g_DI InputsALB.vi"("Action"=T2."read") -> ("DI out"=w41:T3)  [unwired: 10 in]
    n106 = Multiply(x=w20, y=-1.0) -> (x*y=w14:dbl)
    "HandsMotorCmd" <- w14
    n107 = Unbundle By Name(w33) -> ("DIO 0-LiftMinLimitSwitch"=w31:bool, "DIO 2-LiftArmMinLimitSwitch"=w30:bool)
    n108 = Unbundle By Name(w42) -> ("DIO 4-RightArmMaxLimitSwitch"=w52:bool, "DIO 5-RightArmMinLimitSwitch"=w53:bool)
    n109 = Unbundle By Name(w64) -> ("DIO 1-LiftMaxLimitSwitch"=w63:bool, "DIO 3-LiftArmMaxLimitSwitch"=w62:bool)
    n110 = Unbundle By Name(w41) -> ("DIO 6-LeftArmMaxLimitSwitch"=w54:bool, "DIO 7-LeftArmMinLimitSwitch"=w55:bool)
    n111 = Multiply(x=w18, y=-1.0) -> (x*y=w17:dbl)
    n112 = Multiply(x=w23, y=-1.0) -> (x*y=w22:dbl)
    n113 = call <vilib>:"WPI_MotorControlRefNum Registry Get.vi"("refnum name"="HandMotors") -> ("MotorControlDevRef"=w71:T4)  [unwired: 9 in, 1 out]
    n114 = call <vilib>:"WPI_MotorControlRefNum Registry Get.vi"("refnum name"="SqueezeMotor") -> ("MotorControlDevRef"=w28:T4)  [unwired: 9 in, 1 out]
    n115 = call "Drive Command.vi"("X"=w72, "Y"=w22, "Rotation"=w17) -> ()  [unwired: 9 in]
    n116 = call <vilib>:"WPI_MotorControlSetOutput.vi"("Output"=w14, "MotorControlDevRef"=w71) -> ()  [unwired: 7 in, 3 out]
    n117 = call <vilib>:"WPI_MotorControlSetOutput.vi"("Output"=w27, "MotorControlDevRef"=w28) -> ()  [unwired: 7 in, 3 out]
    n118 = Not(x=w31) -> (.not. x?=w34:bool)
    "Lift Max Limit" <- w34
    n119 = Not(x=w63) -> (.not. x?=w67:bool)
    "Arm Lift Max Limit" <- w67
    n120 = Not(x=w54) -> (.not. x?=w46:bool)
    "Left Arm Max Limit" <- w46
    n121 = Not(x=w52) -> (.not. x?=w48:bool)
    "Right Arm Max Limit" <- w48
    n122 = Not(x=w30) -> (.not. x?=w35:bool)
    "Lift Min Limit" <- w35
    n123 = Not(x=w62) -> (.not. x?=w66:bool)
    "Arm Lift Min Limit" <- w66
    n124 = Not(x=w55) -> (.not. x?=w47:bool)
    "Left Arm Min Limit" <- w47
    n125 = Not(x=w53) -> (.not. x?=w49:bool)
    "Right Arm Min Limit" <- w49
    n126 = Multiply(x=w39, y=0.85) -> (x*y=w45:dbl)
    n127 = call "Motor Command with Limit Switches.vi"("LowLimitSwitch"=w35, "MotorCommandIn"=w29, "HighLimitSwitch"=w34) -> (0:w36:dbl)
    "LiftMotorCmd" <- w36
    n128 = call "Motor Command with Limit Switches.vi"("LowLimitSwitch"=w66, "MotorCommandIn"=w60, "HighLimitSwitch"=w67) -> (0:w61:dbl)
    "ArmLiftMotorCmd" <- w61
    n129 = call "Motor Command with Limit Switches.vi"("LowLimitSwitch"=w49, "MotorCommandIn"=w45, "HighLimitSwitch"=w48) -> (0:w51:dbl)
    "RightArmMotorCmd" <- w51
    n130 = call "Motor Command with Limit Switches.vi"("LowLimitSwitch"=w47, "MotorCommandIn"=w45, "HighLimitSwitch"=w46) -> (0:w50:dbl)
    "LeftArmMotorCmd" <- w50
    n131 = call <vilib>:"WPI_MotorControlRefNum Registry Get.vi"("refnum name"="LiftMotor") -> ("MotorControlDevRef"=w37:T4)  [unwired: 9 in, 1 out]
    n132 = call <vilib>:"WPI_MotorControlRefNum Registry Get.vi"("refnum name"="LeftArmMotor") -> ("MotorControlDevRef"=w58:T4)  [unwired: 9 in, 1 out]
    n133 = call <vilib>:"WPI_MotorControlRefNum Registry Get.vi"("refnum name"="ArmLiftMotor") -> ("MotorControlDevRef"=w68:T4)  [unwired: 9 in, 1 out]
    n134 = call <vilib>:"WPI_MotorControlRefNum Registry Get.vi"("refnum name"="RightArmMotor") -> ("MotorControlDevRef"=w59:T4)  [unwired: 9 in, 1 out]
    n135 = call <vilib>:"WPI_MotorControlSetOutput.vi"("Output"=w36, "MotorControlDevRef"=w37) -> ()  [unwired: 7 in, 3 out]
    n136 = call <vilib>:"WPI_MotorControlSetOutput.vi"("Output"=w50, "MotorControlDevRef"=w58) -> ()  [unwired: 7 in, 3 out]
    n137 = call <vilib>:"WPI_MotorControlSetOutput.vi"("Output"=w51, "MotorControlDevRef"=w59) -> ()  [unwired: 7 in, 3 out]
    n138 = call <vilib>:"WPI_MotorControlSetOutput.vi"("Output"=w61, "MotorControlDevRef"=w68) -> ()  [unwired: 7 in, 3 out]
    n139 = Wait (ms)(milliseconds to wait=u32 1 ("millisecond timer value")) -> ()  [unwired: 1 out]
  }
